vi "Error Handler.vi"(3 "Error in":errorcluster) -> (0 "Error out":errorcluster, 1 "Error?":bool)   [LabVIEW 2014, in "Flow Control.lvlib"]
uses:
  <vilib>/Utility/error.llb/DialogType.ctl
  Flow Control.lvlib
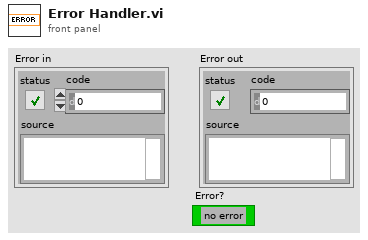
[diagram p1: front panel]
types:
  T1 = typedef "DialogType.ctl" = u16
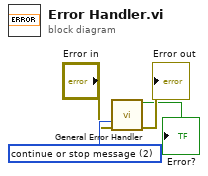
[diagram p0: block diagram]
diagram:
  w4 = T1 2 items=["no dialog", "OK message", "continue or stop message", "OK message + warnings", "continue/stop + warnings"] ("type of dialog (OK msg:1)")
  n1 = call <vilib>:"General Error Handler.vi"("type of dialog (OK msg:1)"=w4, "error in (no error)"="Error in") -> ("error?"=→"Error?":bool, "error out"=→"Error out":errorcluster)  [unwired: 9 in, 3 out]
